vi "rearangeIRDATA-SD.vi"(0 "Brut camera":u32[][](array[numeric])) -> (1 "I channel":u16[][](array[numeric]), 2 "II channel":u16[][](array[numeric]))   [LabVIEW 2015]
panel:
  out "XYgraph":dbl[](graph) caption="Data Values"
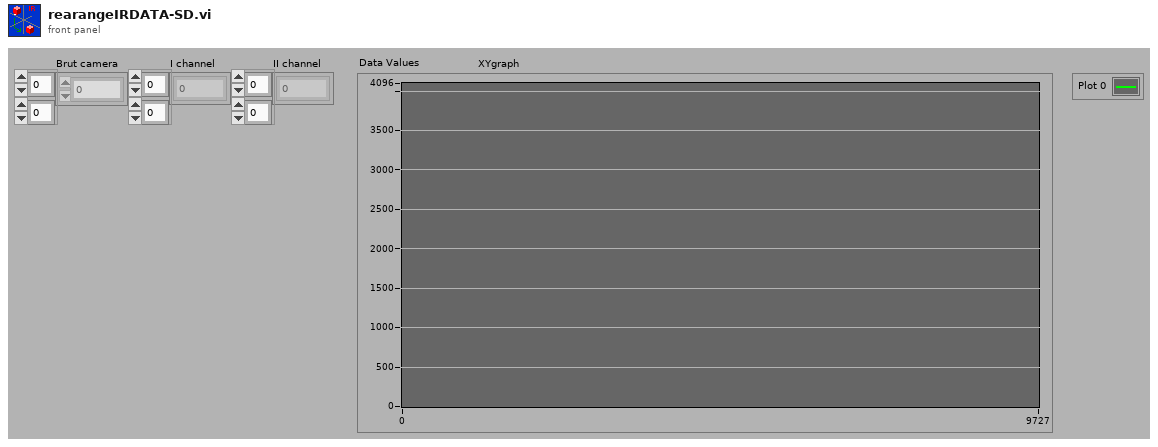
[diagram p1: front panel]
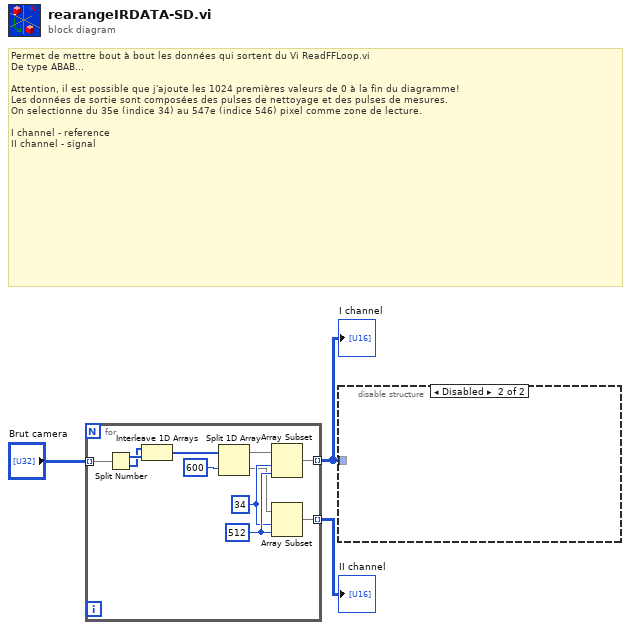
[diagram p0: block diagram]
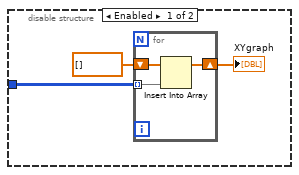
[diagram p2: hidden frame]
diagram:
  # "Permet de mettre bout à bout les données qui sortent du Vi ReadFFLoop.vi\nDe type ABAB...\n\nAttention, il est possible que j'ajoute les 1024 premières valeurs de 0 à la fin du diagramme!\nLes données de sortie sont composées des pulses de nettoyage et des pulses de mesures.\nOn selectionne du 35e (indice 34) au 547e (indice 546) pixel comme zone de lecture.\n\nI channel - reference\nII channel - signal"
  n1 = for {
    tunnel: "Brut camera" -> [w6] mode=indexing
    tunnel: [w5] -> w3 mode=indexing
    tunnel: [w4] -> w2 mode=indexing
    w11 = 34 ("indice")
    w12 = 512 ("longueur")
    n2 = Split Number(x=w6) -> (hi(x)=w8:u16[], lo(x)=w7:u16[])
    n3 = Interleave 1D Arrays(w7, w8) -> (w14:u16[])
    n4 = Split 1D Array(array=w14, index=600 ("indice")) -> (first subarray=w10:u16[], second subarray=w9:u16[])
    n5 = Array Subset(array=w10, index=w11, length=w12) -> (w5:u16[])
    n6 = Array Subset(array=w9, index=w11, length=w12) -> (w4:u16[])
  }
  "I channel" <- w3
  "II channel" <- w2
  n7 = disable-structure shown="Disabled" {
    disable-tunnel: w3 -> [w17 _]
    frame Enabled {
      n8 = for {
        tunnel: w17 -> [w18] mode=indexing
        shift-right: [w19] -> w15
        shift-left: dbl[] [] ("tableau") -> [w20]
        n9 = Insert Into Array(array=w20, new element=w18) -> (w19:dbl[])  [unwired: 1 in]
      }
      "XYgraph" <- w15
    }
    frame Disabled {
    }
  }
